vi "TimeInterpDouble_Clear.vi"(11 "in TimeInterpDouble":T1) -> (3 "out TimeInterpDouble":T1)   [LabVIEW 2019, in "Trajectory_Library.lvlib"]
doc: "Removes all samples from the history buffer.\n\nInputs:\n - In TimeInterpDouble -- Input data cluster.\n\nOutputs:\n - Out TimeInterpDouble -- Updated data cluster."
uses:
  TIME_INTERPOLATABLE_DOUBLE.ctl
  Trajectory_Library.lvlib
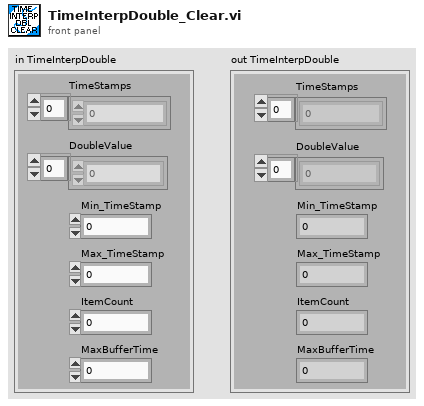
[diagram p1: front panel]
types:
  T1 = typedef "Trajectory_Library.lvlib/TIME_INTERPOLATABLE_DOUBLE.ctl" = cluster{"TimeStamps":dbl[], "DoubleValue":dbl[], "Min_TimeStamp":dbl, "Max_TimeStamp":dbl, "ItemCount":i32, "MaxBufferTime":dbl}
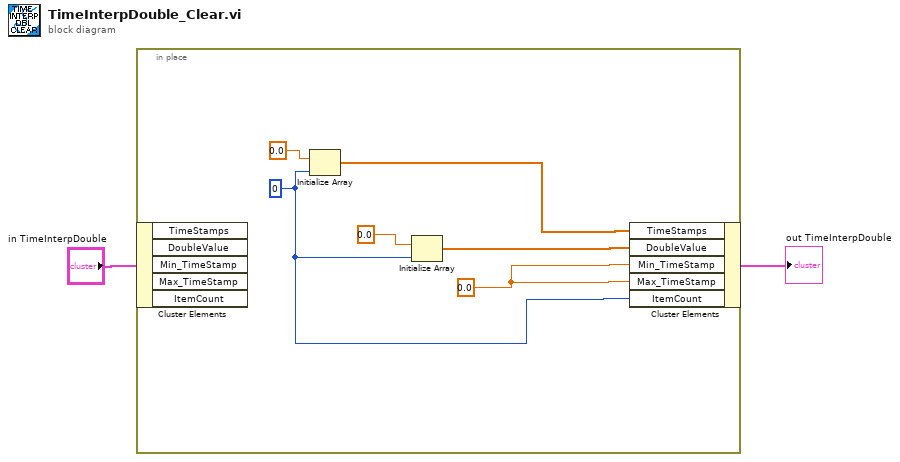
[diagram p0: block diagram]
diagram:
  n1 = in-place {
    w5 = 0.0 ("X")
    w4 = 0 ("dimension size")
    n2 = in-place-cluster #1("in TimeInterpDouble") -> ()  [unwired: 5 out]
    n3 = Initialize Array(0.0 ("element"), w4) -> (w7:dbl[])
    n4 = Initialize Array(0.0 ("element"), w4) -> (w6:dbl[])
    n5 = in-place-cluster #1("TimeStamps"=w7, "DoubleValue"=w6, "Min_TimeStamp"=w5, "Max_TimeStamp"=w5, "ItemCount"=w4) -> (→"out TimeInterpDouble":T1)
  }
